vi "Options.vi"(7 "Read?":bool=TRUE, 11 "Options":T1={"Color"=16723218, "pen"={"Width"=2, "Style"=enum."Solid"}, "font"={"Font Name"="Arial", "Size"=14, "Strikeout?"=FALSE, "Italic?"=FALSE, "Underline?"=FALSE, "Outline?"=FALSE, "Shadow?"=FALSE, "Bold?"=FALSE, "FontColor"=6908265}, "caption"="Click to set a point marker"}) -> (3 "Options out":T1={"Color"=16723218, "pen"={"Width"=2, "Style"=enum."Solid"}, "font"={"Font Name"="Arial", "Size"=14, "Strikeout?"=FALSE, "Italic?"=FALSE, "Underline?"=FALSE, "Outline?"=FALSE, "Shadow?"=FALSE, "Bold?"=FALSE, "FontColor"=6908265}, "caption"="Click to set a point marker"})   [LabVIEW 2020, in "Graph Extensions.lvlib"]
uses:
  Graph Extensions.lvlib
  controls/MarkerOptions.ctl
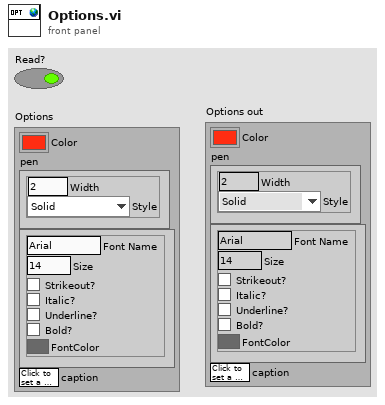
[diagram p1: front panel]
types:
  T1 = typedef "Graph Extensions.lvlib/MarkerOptions.ctl" = cluster{"Color":u32, "pen":cluster{"Width":u16, "Style":enum32{"Solid", "Dash", "Dot", "DashDot", "DashDotDot"}}, "font":cluster{"Font Name":string, "Size":i16, "Strikeout?":bool, "Italic?":bool, "Underline?":bool, "Outline?":bool, "Shadow?":bool, "Bold?":bool, "FontColor":u32}, "caption":string}
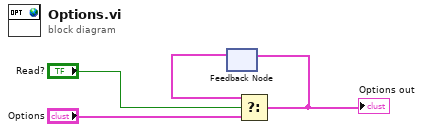
[diagram p0: block diagram]
diagram:
  n1 = feedback #1() -> (w1:T1)  [unwired: 1 in]
  n2 = Select(t=w1, s="Read?", f="Options") -> (s? t:f=w2:T1)
  "Options out" <- w2
  n3 = feedback-in #1(w2) -> ()
